vi "SVT Initialize Swept Sine (DAQmx).vi"(7 "AO source settings":T7={"excitation channel"="ao0", "max value [V]"=10.0, "min value [V]"=-10.0, "terminal configuration"=-1} {"terminal configuration" items=["Default"=-1, "RSE"=10083, "Differential"=10106, "Pseudodifferential"=12529]; "min value [V]" format="%0.2f"; "max value [V]" format="%0.2f"}, 8 "error in (no error)":errorcluster, 9 "AI response settings":T5={"response channel"="ai1", "max value [V]"=10.0, "min value [V]"=-10.0, "terminal configuration"=-1} {"terminal configuration" items=["Default"=-1, "RSE"=10083, "NRSE"=10078, "Differential"=10106, "Pseudodifferential"=12529]; "min value [V]" format="%.2f"; "max value [V]" format="%.2f"}, 10 "AI stimulus settings":T6={"stimulus channel"="ai0", "max value [V]"=10.0, "min value [V]"=-10.0, "terminal configuration"=-1} {"terminal configuration" items=["Default"=-1, "RSE"=10083, "NRSE"=10078, "Differential"=10106, "Pseudodifferential"=12529]; "min value [V]" format="%.2f"; "max value [V]" format="%.2f"}, 11 "DAQmx device":tag) -> (0 "error out":errorcluster, 2 "device name":string, 3 "swept sine task out":T1={"source settings"={"AO task name"="", "source"=[]}, "stimulus settings"={"stimulus task name"="", "stimulus"=[]}, "response(s) settings"={"response task name"="", "response"=[]}, "measurement settings"={"AI sampling frequency"=51200.0, "AO sampling frequency"=1024.0, "AI block size"=1024, "AO block Size"=1024, "block duration [ms]"=0.0, "number of AI channels"=0, "device propagation delay [samples]"=0.0, "total propagation time [samples]"=0.0, "DUT propagation time [ms]"=0.0}, "linlog"=enum."linear", "repeat"=enum."off", "frequency list"=[1.0], "amplitude list"=[1.0], "settling time"={"settle time"=0.015599999576807022, "settle cycles"=5}, "integration time"={"integration time"=0.015599999576807022, "integration cycles"=5}, "frequencies indices"={"AI freq index"=0, "AO freq index"=5}, "read marks"={"write index"=0, "read index"=0, "freq start index"=0, "freq stop index"=0, "# extracted"=0, "buffer type"=enum."Invalid buffer", "read/write indices"=[], "AO index"=0, "AI index"=0, "settled"=FALSE, "integration done"=FALSE}, "harmonic settings"={"maximum THD harmonic"=5, "harmonic mapping"=[1], "units"={"THD unit"=enum."%", "nth harmonic unit"=enum."%", "SINAD unit"=enum."dB", "THD+N unit"=enum."dB"}}, "auto resolution settings"={"auto max step"=512, "slow threshold db"=6.0, "fast threshold db"=1.0}, "auto level settings"={"auto level enable"=FALSE, "auto level channel"=6, "ideal ref"=1.0, "max level"=10.0, "ref upper deviation db"=3.0, "ref lower deviation db"=-3.0}, "offset"=1.0, "ramping rate"=0.0, "phase"=0.0, "initialize"=FALSE} {"phase" format="%.2f"; "response(s) settings"."response"."channel info"."pregain" format="%.2f"; "response(s) settings"."response"."channel info"."weighting filter" items=["Linear", "A-weighting", "B-weighting", "C-weighting", "ITU-R 468-4", "Dolby", "CCITT", "C-message", "Wb", "Wc", "Wd", "We", "Wf", "Wh", "Wj", "Wk", "Wm", "AES17 20 kHz lowpass", "AES17 40 kHz lowpass", "AES17 20 kHz highpass", "AES17 40 kHz highpass"]; "response(s) settings"."response"."channel info"."dB reference" format="%^.1e"; "response(s) settings"."response"."channel info"."engineering units" items=["custom..."=0, "V"=1, "A"=21, "C"=30, "pC"=31, "s"=32, "-"=29, "Pa"=2, "N"=20, "g"=3, "m/s^2"=4, "m/s"=5, "m"=6, "mm/s"=12, "mm"=13, "micron/s"=14, "micron"=15, "in/s^2"=7, "in/s"=8, "in"=9, "mil/s"=10, "mil"=11, "rad/s^2"=16, "rad/s"=17, "rad"=18, "deg/s^2"=26, "deg/s"=27, "deg"=28, "RPM"=22, "cycle/s^2"=23, "Hz"=24, "cycle"=25, "strain"=19]; "response(s) settings"."response"."channel info"."sensor sensitivity" format="%#_5f"; "stimulus settings"."stimulus"."channel info"."pregain" format="%.2f"; "stimulus settings"."stimulus"."channel info"."weighting filter" items=["Linear", "A-weighting", "B-weighting", "C-weighting", "ITU-R 468-4", "Dolby", "CCITT", "C-message", "Wb", "Wc", "Wd", "We", "Wf", "Wh", "Wj", "Wk", "Wm", "AES17 20 kHz lowpass", "AES17 40 kHz lowpass", "AES17 20 kHz highpass", "AES17 40 kHz highpass"]; "stimulus settings"."stimulus"."channel info"."dB reference" format="%^.1e"; "stimulus settings"."stimulus"."channel info"."engineering units" items=["custom..."=0, "V"=1, "A"=21, "C"=30, "pC"=31, "s"=32, "-"=29, "Pa"=2, "N"=20, "g"=3, "m/s^2"=4, "m/s"=5, "m"=6, "mm/s"=12, "mm"=13, "micron/s"=14, "micron"=15, "in/s^2"=7, "in/s"=8, "in"=9, "mil/s"=10, "mil"=11, "rad/s^2"=16, "rad/s"=17, "rad"=18, "deg/s^2"=26, "deg/s"=27, "deg"=28, "RPM"=22, "cycle/s^2"=23, "Hz"=24, "cycle"=25, "strain"=19]; "stimulus settings"."stimulus"."channel info"."sensor sensitivity" format="%#_5f"; "ramping rate" format="%.4f"; "offset" format="%.2f"; "auto level settings"."ref lower deviation db" format="%.4f"; "auto level settings"."ref upper deviation db" format="%.4f"; "auto level settings"."max level" format="%.4f"; "auto level settings"."ideal ref" format="%.4f"; "auto resolution settings"."fast threshold db" format="%.4f"; "auto resolution settings"."slow threshold db" format="%.4f"; "harmonic settings"."maximum THD harmonic" max=10 step=1; "integration time"."integration time" format="%.2p"; "settling time"."settle time" format="%.2p"; "amplitude list" format="%.2f"; "frequency list" format="%.2f"; "measurement settings"."DUT propagation time [ms]" format="%.2f"; "measurement settings"."AO sampling frequency" format="%.2f"; "measurement settings"."AI sampling frequency" format="%.2f"})   [LabVIEW 2017]
doc: "Initializes swept-sine-analysis parameters on analog input and output devices."
uses:
  <vilib>/addons/Sound and Vibration/svt_Swept Sine/subVIs/sv_Swept Sine Task.ctl
  <vilib>/addons/_NISVFA/_Shared subVIs/Controls/svc_Channel Info.ctl
  <vilib>/addons/_NISVFA/_Shared subVIs/Controls/svc_Engineering Units Text Ring.ctl
  <vilib>/addons/_NISVFA/_Shared subVIs/Controls/svc_Weighting Filter Text Ring.ctl
  <vilib>/DAQmx/create/channels.llb/DAQmx Create Channel (AI-Voltage-Basic).vi
  <vilib>/DAQmx/create/channels.llb/DAQmx Create Channel (AO-Voltage-Basic).vi
  <resource>/objmgr/daqmx.rc
  <vilib>/addons/Sound and Vibration/svt_Swept Sine/SoundVib_SweptSine.lvlib
panel:
  in  "swept sine task default":T1={"source settings"={"AO task name"="", "source"=[]}, "stimulus settings"={"stimulus task name"="", "stimulus"=[]}, "response(s) settings"={"response task name"="", "response"=[]}, "measurement settings"={"AI sampling frequency"=51200.0, "AO sampling frequency"=51200.0, "AI block size"=1024, "AO block Size"=0, "block duration [ms]"=1024.0, "number of AI channels"=0, "device propagation delay [samples]"=0.0, "total propagation time [samples]"=0.0, "DUT propagation time [ms]"=0.0}, "linlog"=enum."linear", "repeat"=enum."off", "frequency list"=[1.0], "amplitude list"=[1.0], "settling time"={"settle time"=0.015599999576807022, "settle cycles"=5}, "integration time"={"integration time"=0.015599999576807022, "integration cycles"=5}, "frequencies indices"={"AI freq index"=0, "AO freq index"=0}, "read marks"={"write index"=0, "read index"=0, "freq start index"=0, "freq stop index"=0, "# extracted"=0, "buffer type"=enum."Invalid buffer", "read/write indices"=[], "AO index"=0, "AI index"=0, "settled"=FALSE, "integration done"=FALSE}, "harmonic settings"={"maximum THD harmonic"=5, "harmonic mapping"=[1], "units"={"THD unit"=enum."%", "nth harmonic unit"=enum."%", "SINAD unit"=enum."dB", "THD+N unit"=enum."dB"}}, "auto resolution settings"={"auto max step"=512, "slow threshold db"=6.0, "fast threshold db"=1.0}, "auto level settings"={"auto level enable"=FALSE, "auto level channel"=0, "ideal ref"=1.0, "max level"=10.0, "ref upper deviation db"=3.0, "ref lower deviation db"=-3.0}, "offset"=1.0, "ramping rate"=0.0, "phase"=0.0, "initialize"=FALSE} {"phase" format="%.2f"; "response(s) settings"."response"."channel info"."pregain" format="%.2f"; "response(s) settings"."response"."channel info"."weighting filter" items=["Linear", "A-weighting", "B-weighting", "C-weighting", "ITU-R 468-4", "Dolby", "CCITT", "C-message", "Wb", "Wc", "Wd", "We", "Wf", "Wh", "Wj", "Wk", "Wm", "AES17 20 kHz lowpass", "AES17 40 kHz lowpass", "AES17 20 kHz highpass", "AES17 40 kHz highpass"]; "response(s) settings"."response"."channel info"."dB reference" format="%^.1e"; "response(s) settings"."response"."channel info"."engineering units" items=["custom..."=0, "V"=1, "A"=21, "C"=30, "pC"=31, "s"=32, "-"=29, "Pa"=2, "N"=20, "g"=3, "m/s^2"=4, "m/s"=5, "m"=6, "mm/s"=12, "mm"=13, "micron/s"=14, "micron"=15, "in/s^2"=7, "in/s"=8, "in"=9, "mil/s"=10, "mil"=11, "rad/s^2"=16, "rad/s"=17, "rad"=18, "deg/s^2"=26, "deg/s"=27, "deg"=28, "RPM"=22, "cycle/s^2"=23, "Hz"=24, "cycle"=25, "strain"=19]; "response(s) settings"."response"."channel info"."sensor sensitivity" format="%#_5f"; "stimulus settings"."stimulus"."channel info"."pregain" format="%.2f"; "stimulus settings"."stimulus"."channel info"."weighting filter" items=["Linear", "A-weighting", "B-weighting", "C-weighting", "ITU-R 468-4", "Dolby", "CCITT", "C-message", "Wb", "Wc", "Wd", "We", "Wf", "Wh", "Wj", "Wk", "Wm", "AES17 20 kHz lowpass", "AES17 40 kHz lowpass", "AES17 20 kHz highpass", "AES17 40 kHz highpass"]; "stimulus settings"."stimulus"."channel info"."dB reference" format="%^.1e"; "stimulus settings"."stimulus"."channel info"."engineering units" items=["custom..."=0, "V"=1, "A"=21, "C"=30, "pC"=31, "s"=32, "-"=29, "Pa"=2, "N"=20, "g"=3, "m/s^2"=4, "m/s"=5, "m"=6, "mm/s"=12, "mm"=13, "micron/s"=14, "micron"=15, "in/s^2"=7, "in/s"=8, "in"=9, "mil/s"=10, "mil"=11, "rad/s^2"=16, "rad/s"=17, "rad"=18, "deg/s^2"=26, "deg/s"=27, "deg"=28, "RPM"=22, "cycle/s^2"=23, "Hz"=24, "cycle"=25, "strain"=19]; "stimulus settings"."stimulus"."channel info"."sensor sensitivity" format="%#_5f"; "ramping rate" format="%.4f"; "offset" format="%.2f"; "auto level settings"."ref lower deviation db" format="%.4f"; "auto level settings"."ref upper deviation db" format="%.4f"; "auto level settings"."max level" format="%.4f"; "auto level settings"."ideal ref" format="%.4f"; "auto resolution settings"."fast threshold db" format="%.4f"; "auto resolution settings"."slow threshold db" format="%.4f"; "harmonic settings"."maximum THD harmonic" max=10 step=1; "integration time"."integration time" format="%.2p"; "settling time"."settle time" format="%.2p"; "amplitude list" format="%.2f"; "frequency list" format="%.2f"; "measurement settings"."DUT propagation time [ms]" format="%.2f"; "measurement settings"."AO sampling frequency" format="%.2f"; "measurement settings"."AI sampling frequency" format="%.2f"}
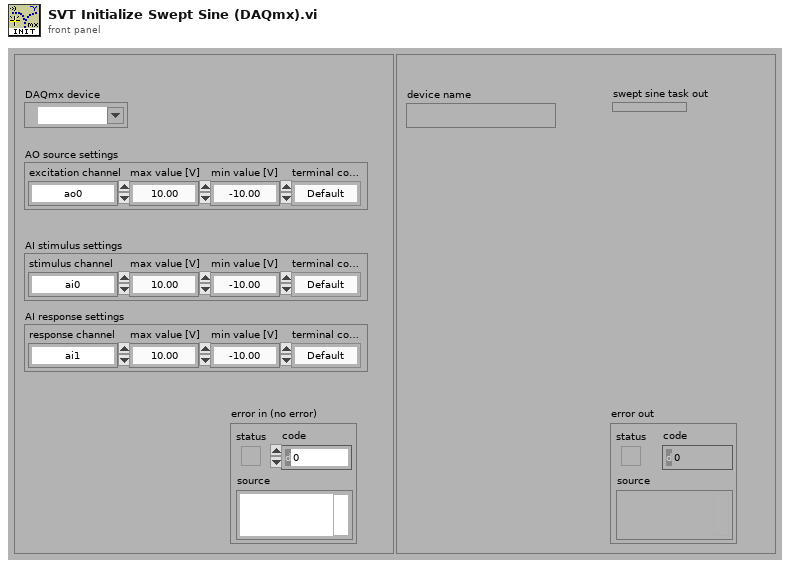
[diagram p1: front panel]
types:
  T1 = typedef "SoundVib_SweptSine.lvlib/sv_Swept Sine Task.ctl" = cluster{"source settings":cluster{"AO task name":refnum<k21>, "source":cluster{"AO physical channel":tag}[]}, "stimulus settings":cluster{"stimulus task name":refnum<k21>, "stimulus":cluster{"stimulus physical channel":tag, "channel info":T2}[]}, "response(s) settings":cluster{"response task name":refnum<k21>, "response":cluster{"response physical channel":tag, "channel info":T2}[]}, "measurement settings":cluster{"AI sampling frequency":dbl, "AO sampling frequency":dbl, "AI block size":i32, "AO block Size":i32, "block duration [ms]":dbl, "number of AI channels":i32, "device propagation delay [samples]":dbl, "total propagation time [samples]":dbl, "DUT propagation time [ms]":dbl}, "linlog":enum16{"linear", "log"}, "repeat":enum16{"off", "on"}, "frequency list":dbl[], "amplitude list":dbl[], "settling time":cluster{"settle time":dbl, "settle cycles":i32}, "integration time":cluster{"integration time":dbl, "integration cycles":i32}, "frequencies indices":cluster{"AI freq index":i32, "AO freq index":i32}, "read marks":cluster{"write index":u32, "read index":u32, "freq start index":u32, "freq stop index":u32, "# extracted":u32, "buffer type":enum16{"Invalid buffer", "Intermediate buffer", "Final buffer"}, "read/write indices":cluster{"settle time index":u32, "integration time index":u32}[], "AO index":i32, "AI index":i32, "settled":bool, "integration done":bool}, "harmonic settings":cluster{"maximum THD harmonic":u32, "harmonic mapping":u32[], "units":cluster{"THD unit":enum16{"dB", "%"}, "nth harmonic unit":enum16{"dB", "%"}, "SINAD unit":enum16{"dB", "%"}, "THD+N unit":enum16{"dB", "%"}}}, "auto resolution settings":cluster{"auto max step":i32, "slow threshold db":dbl, "fast threshold db":dbl}, "auto level settings":cluster{"auto level enable":bool, "auto level channel":u8, "ideal ref":sgl, "max level":sgl, "ref upper deviation db":sgl, "ref lower deviation db":sgl}, "offset":dbl, "ramping rate":dbl, "phase":dbl, "initialize":bool}
  T2 = typedef "svc_Channel Info.ctl" = cluster{"sensor sensitivity":dbl, "engineering units":T3, "dB reference":dbl, "custom label":string, "weighting filter":T4, "pregain":dbl}
  T3 = typedef "svc_Engineering Units Text Ring.ctl" = u16
  T4 = typedef "svc_Weighting Filter Text Ring.ctl" = u16
  T5 = cluster{"response channel":string, "max value [V]":dbl, "min value [V]":dbl, "terminal configuration":i32}
  T6 = cluster{"stimulus channel":string, "max value [V]":dbl, "min value [V]":dbl, "terminal configuration":i32}
  T7 = cluster{"excitation channel":string, "max value [V]":dbl, "min value [V]":dbl, "terminal configuration":i32}
  T8 = cluster{"settle time index":u32, "integration time index":u32}[]
  T9 = enum16{"Invalid buffer", "Intermediate buffer", "Final buffer"}
  T10 = cluster{"DAQmx Physical Channel":tag, "channel info":T2}
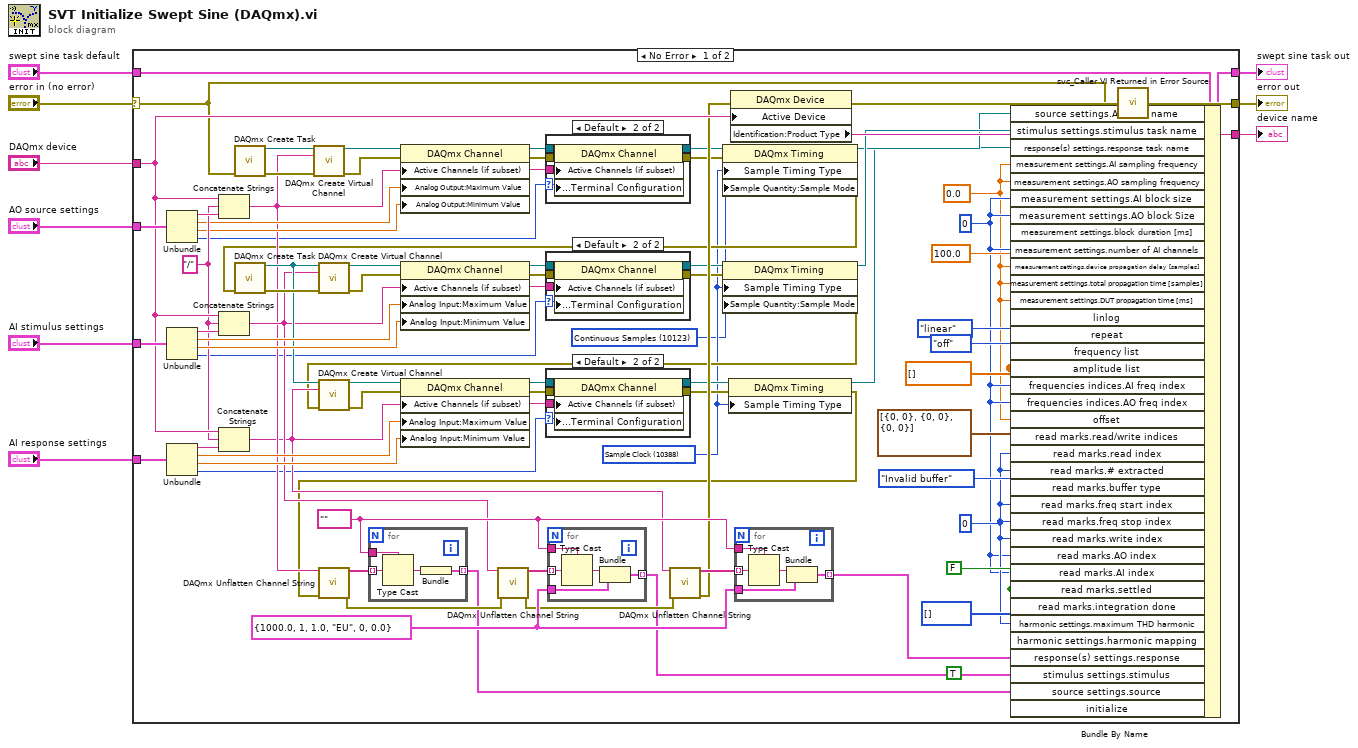
[diagram p0: block diagram]
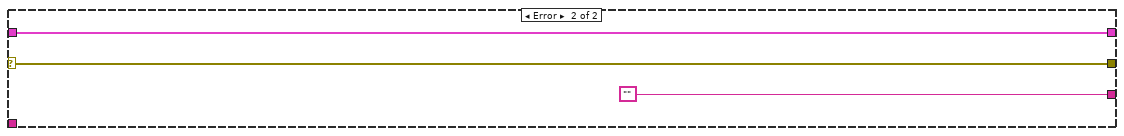
[diagram p5: hidden frame]
diagram:
  n1 = case shown="No Error" "error in (no error)" {
    selector: "error in (no error)" -> [w11 w129]
    tunnel: [w81 w129] -> w8
    tunnel: [w78 w127] -> w7
    tunnel: "AO source settings" -> [w63 _]
    tunnel: "AI stimulus settings" -> [w72 _]
    tunnel: "AI response settings" -> [w67 _]
    tunnel: "DAQmx device" -> [w62 _]
    tunnel: [w43 ""] -> w6
    tunnel: "swept sine task default" -> [w80 w127]
    frame No Error {
      w52 = T2 {"sensor sensitivity"=1000.0, "engineering units"=1, "dB reference"=1.0, "custom label"="EU", "weighting filter"=0, "pregain"=0.0} ("channel info")
      w86 = dbl[] [] ("frequency list")
      w38 = 0.0 ("measurement settings.AI sampling frequency")
      w10 = 10123 items=["Finite Samples"=10178, "Continuous Samples"=10123, "Hardware Timed Single Point"=12522] ("SampQuant.SampMode")
      w13 = 10388 items=["Sample Clock"=10388, "Handshake"=10389, "Implicit"=10451, "On Demand"=10390, "Change Detection"=12504] ("SampTimingType")
      w42 = 0 ("AO device settings.AO Settings.AO taskID")
      w49 = tag "" ("DAQmx Physical Channel")
      w61 = "/" ("string")
      w84 = FALSE ("acq state.settled")
      w79 = u32 0 ("AO device settings.AO Settings.AO taskID")
      n2 = Unbundle(w63) -> ("excitation channel"=w64:string, "max value [V]"=w58:dbl, "min value [V]"=w57:dbl, "terminal configuration"=w28:i32)
      n3 = Unbundle(w72) -> ("stimulus channel"=w76:string, "max value [V]"=w66:dbl, "min value [V]"=w73:dbl, "terminal configuration"=w27:i32)
      n4 = Unbundle(w67) -> ("response channel"=w68:string, "max value [V]"=w65:dbl, "min value [V]"=w71:dbl, "terminal configuration"=w26:i32)
      n5 = Concatenate Strings(w62, w61, w64) -> (w30:string)
      n6 = Concatenate Strings(w62, w61, w76) -> (w31:string)
      n7 = Concatenate Strings(w62, w61, w68) -> (w29:string)
      n8 = call <vilib>:"DAQmx Create Task.vi"("error in"=w11) -> ("task out"=w77:refnum<k21>, "error out"=w51:errorcluster)  [unwired: 13 in]
      n9 = call-poly <vilib>:"DAQmx Create Virtual Channel.vi"("task in"=w77, "physical channels"=w30, "error in"=w51) -> ("task out"=w60:refnum<k21>, "error out"=w59:errorcluster)  [unwired: 11 in]
      n10 = property class="DAQmx Channel"(reference=w60, error in=w59, "Active Channels (if subset)"=w30, "Analog Output:Maximum Value"=w58, "Analog Output:Minimum Value"=w57) -> (reference out=w37:refnum<k21>, error out=w36:errorcluster)
      n11 = case shown="Default" w28 {
        selector: w28 -> [_ w107]
        tunnel: w37 -> [w106 w112]
        tunnel: w36 -> [w105 w111]
        tunnel: [w106 w110] -> w22
        tunnel: w30 -> [_ w109]
        tunnel: [w105 w108] -> w18
        frame -1 {
          # "Use default:\nterminal config"
        }
        frame Default {
          n12 = property class="DAQmx Channel"(reference=w112, error in=w111, "Active Channels (if subset)"=w109, "Analog Output:General Properties:Output Configuration:Terminal Configuration"=w107) -> (reference out=w110:refnum<k21>, error out=w108:errorcluster)
        }
      }
      n13 = property class="DAQmx Timing"(reference=w22, error in=w18, "Sample Timing Type"=w13, "Sample Quantity:Sample Mode"=w10) -> (reference out=w23:refnum<k21>, error out=w19:errorcluster)
      n14 = call <vilib>:"DAQmx Create Task.vi"("error in"=w19) -> ("task out"=w48:refnum<k21>, "error out"=w50:errorcluster)  [unwired: 13 in]
      n15 = call-poly <vilib>:"DAQmx Create Virtual Channel.vi"("task in"=w48, "physical channels"=w31, "error in"=w50) -> ("task out"=w74:refnum<k21>, "error out"=w75:errorcluster)  [unwired: 11 in]
      n16 = property class="DAQmx Channel"(reference=w74, error in=w75, "Active Channels (if subset)"=w31, "Analog Input:Maximum Value"=w66, "Analog Input:Minimum Value"=w73) -> (reference out=w35:refnum<k21>, error out=w34:errorcluster)
      n17 = case shown="Default" w27 {
        selector: w27 -> [_ w99]
        tunnel: w35 -> [w98 w104]
        tunnel: w34 -> [w97 w103]
        tunnel: [w98 w102] -> w24
        tunnel: w31 -> [_ w101]
        tunnel: [w97 w100] -> w16
        frame -1 {
          # "Use default:\nterminal config"
        }
        frame Default {
          n18 = property class="DAQmx Channel"(reference=w104, error in=w103, "Active Channels (if subset)"=w101, "Analog Input:General Properties:Input Configuration:Terminal Configuration"=w99) -> (reference out=w102:refnum<k21>, error out=w100:errorcluster)
        }
      }
      n19 = property class="DAQmx Timing"(reference=w24, error in=w16, "Sample Timing Type"=w13, "Sample Quantity:Sample Mode"=w10) -> (reference out=w25:refnum<k21>, error out=w17:errorcluster)
      n20 = call-poly <vilib>:"DAQmx Create Virtual Channel.vi"("task in"=w48, "physical channels"=w29, "error in"=w17) -> ("task out"=w70:refnum<k21>, "error out"=w69:errorcluster)  [unwired: 11 in]
      n21 = property class="DAQmx Channel"(reference=w70, error in=w69, "Active Channels (if subset)"=w29, "Analog Input:Maximum Value"=w65, "Analog Input:Minimum Value"=w71) -> (reference out=w33:refnum<k21>, error out=w32:errorcluster)
      n22 = case shown="Default" w26 {
        selector: w26 -> [_ w91]
        tunnel: w33 -> [w90 w96]
        tunnel: w32 -> [w89 w95]
        tunnel: [w90 w94] -> w20
        tunnel: w29 -> [_ w93]
        tunnel: [w89 w92] -> w14
        frame -1 {
          # "Use default:\nterminal config"
        }
        frame Default {
          n23 = property class="DAQmx Channel"(reference=w96, error in=w95, "Active Channels (if subset)"=w93, "Analog Input:General Properties:Input Configuration:Terminal Configuration"=w91) -> (reference out=w94:refnum<k21>, error out=w92:errorcluster)
        }
      }
      n24 = property class="DAQmx Timing"(reference=w20, error in=w14, "Sample Timing Type"=w13) -> (reference out=w21:refnum<k21>, error out=w15:errorcluster)
      n25 = call <vilib>:"DAQmx Unflatten Channel String.vi"("names in"=w30, "error in"=w15) -> ("names out"=w56:string[], "error out"=w47:errorcluster)  [unwired: 12 in]
      n26 = for {
        tunnel: w56 -> [w125] mode=indexing
        tunnel: [w126] -> w41 mode=indexing
        tunnel: w49 -> [w123]
        n27 = Type Cast(type=w123, x=w125) -> (*(type *) &x=w124:tag)
        n28 = Bundle("DAQmx Physical Channel"=w124) -> (w126:cluster{"DAQmx Physical Channel":tag})  [unwired: 1 in]
      }
      n29 = call <vilib>:"DAQmx Unflatten Channel String.vi"("names in"=w31, "error in"=w47) -> ("names out"=w55:string[], "error out"=w46:errorcluster)  [unwired: 12 in]
      n30 = for {
        tunnel: w55 -> [w121] mode=indexing
        tunnel: [w122] -> w40 mode=indexing
        tunnel: w49 -> [w119]
        tunnel: w52 -> [w118]
        n31 = Type Cast(type=w119, x=w121) -> (*(type *) &x=w120:tag)
        n32 = Bundle("DAQmx Physical Channel"=w120, "channel info"=w118) -> (w122:T10)  [unwired: 1 in]
      }
      n33 = call <vilib>:"DAQmx Unflatten Channel String.vi"("names in"=w29, "error in"=w46) -> ("names out"=w53:string[], "error out"=w45:errorcluster)  [unwired: 12 in]
      n34 = property class="DAQmx Device"(error in=w45, "Active Device"=w62) -> (error out=w44:errorcluster, "Identification:Product Type"=w43:string)  [unwired: 1 in, 1 out]
      n35 = for {
        tunnel: w53 -> [w116] mode=indexing
        tunnel: [w117] -> w39 mode=indexing
        tunnel: w49 -> [w114]
        tunnel: w52 -> [w113]
        n36 = Type Cast(type=w114, x=w116) -> (*(type *) &x=w115:tag)
        n37 = Bundle("DAQmx Physical Channel"=w115, "channel info"=w113) -> (w117:T10)  [unwired: 1 in]
      }
      n38 = Bundle By Name(cluster=w80, "source settings.AO task name"=w23, "stimulus settings.stimulus task name"=w25, "response(s) settings.response task name"=w21, "measurement settings.AI sampling frequency"=w38, "measurement settings.AO sampling frequency"=w38, "measurement settings.AI block size"=w42, "measurement settings.AO block Size"=w42, "measurement settings.block duration [ms]"=100.0, "measurement settings.number of AI channels"=w42, "measurement settings.device propagation delay [samples]"=w38, "measurement settings.total propagation time [samples]"=w38, "measurement settings.DUT propagation time [ms]"=w38, "linlog"=enum16{"linear", "log"}."linear", "repeat"=enum16{"off", "on"}."off", "frequency list"=w86, "amplitude list"=w86, "frequencies indices.AI freq index"=w42, "frequencies indices.AO freq index"=w42, "offset"=w38, "read marks.read/write indices"=T8 [{"settle time index"=0, "integration time index"=0}, {"settle time index"=0, "integration time index"=0}, {"settle time index"=0, "integration time index"=0}] ("initialized array"), "read marks.read index"=w79, "read marks.# extracted"=w79, "read marks.buffer type"=T9."Invalid buffer", "read marks.freq start index"=w79, "read marks.freq stop index"=w79, "read marks.write index"=w79, "read marks.AO index"=w42, "read marks.AI index"=w42, "read marks.settled"=w84, "read marks.integration done"=w84, "harmonic settings.maximum THD harmonic"=w79, "harmonic settings.harmonic mapping"=u32[] [], "response(s) settings.response"=w39, "stimulus settings.stimulus"=w40, "source settings.source"=w41, "initialize"=TRUE) -> (w78:T1)
      n39 = call <vilib>:"svc_Caller VI Returned in Error Source.vi"("warning input to caller"=w11, "error in (no error)"=w44) -> ("error out"=w81:errorcluster)  [unwired: 3 in]
    }
    frame Error {
    }
  }
  "error out" <- w8
  "swept sine task out" <- w7
  "device name" <- w6
